vi "In Range.vi"(2 "Tolerance":dbl, 3 "2":dbl, 4 "1":dbl) -> (0 "Results":bool)   [LabVIEW 2019]
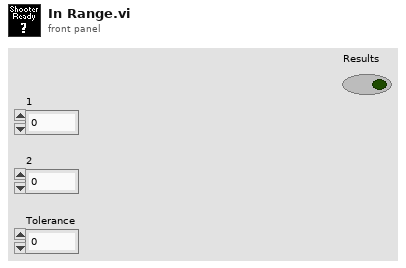
[diagram p1: front panel]
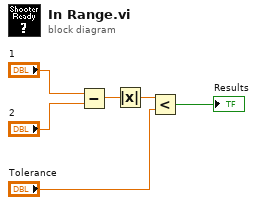
[diagram p0: block diagram]
diagram:
  n1 = Subtract(x="1", y="2") -> (x-y=w4:dbl)
  n2 = Absolute Value(x=w4) -> (abs(x)=w3:dbl)
  n3 = Less?(x=w3, y="Tolerance") -> (x < y?=→"Results":bool)
